vi "Sel_Insert QuickDrop.vi"(6 "Variant in":variant, 7 "Shift Pressed?":bool, 8 "error in (no error)":errorcluster, 10 "QD Combo Box Ref":refnum<vi>, 11 "QD Launch VI Ref":refnum<vi>) -> (0 "error out":errorcluster, 4 "Variant out":variant)   [LabVIEW 2014]
doc: "This quickdrop functionality will insert the selected node in the selected wire. Make sure that selected wire and node terminals have same data type.\n\nDefault Shortcut - [`]"
panel:
  in  "Undo Name":string="Quick Drop Keyboard Shortcut"
  # "Do not change the connector pane of this VI.\n\nSee the block diagram for directions on how to use this template."
  # "Specify the name of the Undo transaction"
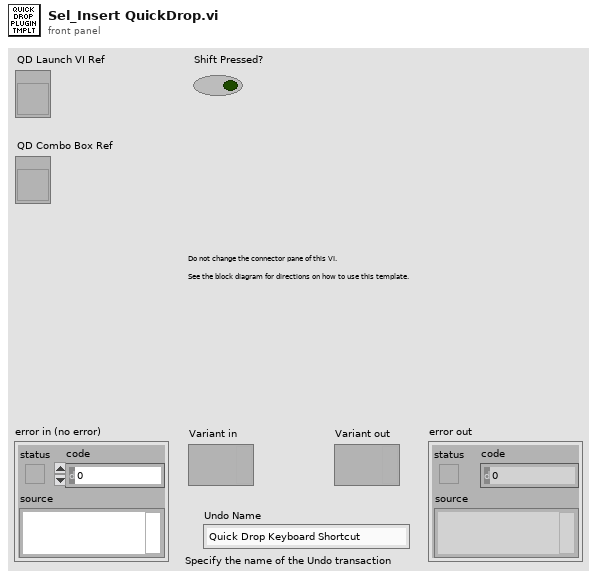
[diagram p1: front panel]
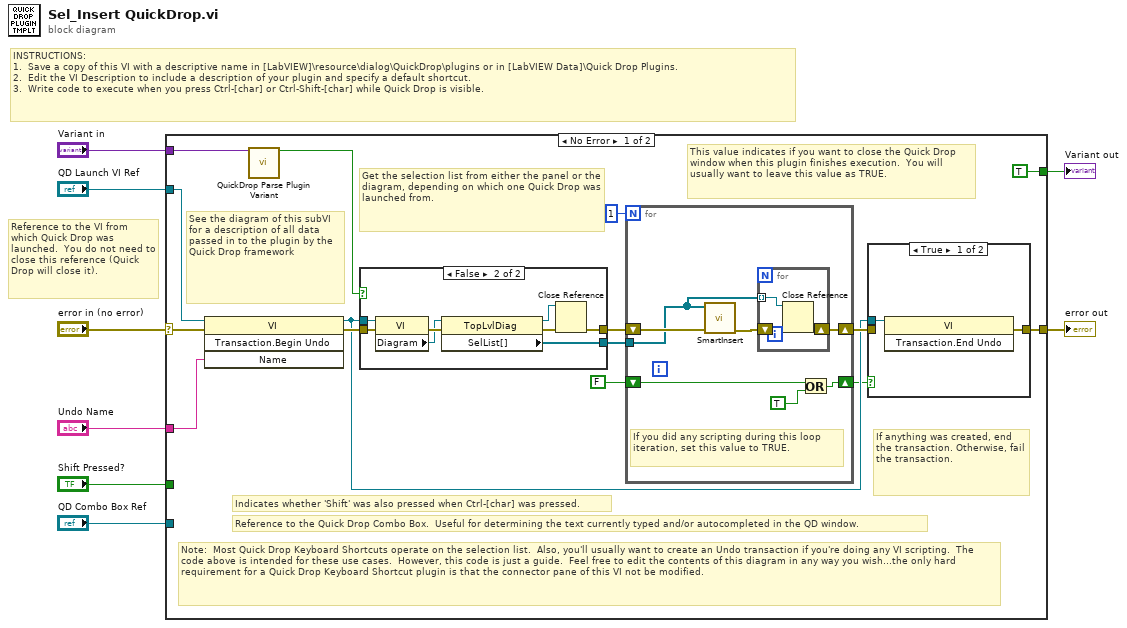
[diagram p0: block diagram]
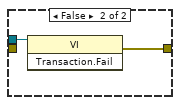
[diagram p2: hidden frame]
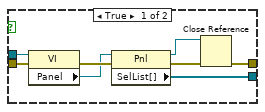
[diagram p3: hidden frame]
diagram:
  # "Reference to the VI from which Quick Drop was launched.  You do not need to close this reference (Quick Drop will close it)."
  # "INSTRUCTIONS:\n1.  Save a copy of this VI with a descriptive name in [LabVIEW]\\resource\\dialog\\QuickDrop\\plugins or in [LabVIEW Data]\\Quick Drop Plugins.\n2.  Edit the VI Description to include a description of your plugin and specify a default shortcut. \n3.  Write code to execute when you press Ctrl-[char] or Ctrl-Shift-[char] while Quick Drop is visible."
  n1 = case shown="No Error" "error in (no error)" {
    selector: "error in (no error)" -> [w22 w54]
    tunnel: [w16 w54] -> w7
    tunnel: "QD Launch VI Ref" -> [w21 _]
    tunnel: "Shift Pressed?" -> [_ _]
    tunnel: "QD Combo Box Ref" -> [_ _]
    tunnel: "Variant in" -> [w23 _]
    tunnel: "Undo Name" -> [w20 _]
    tunnel: [TRUE _] -> w1
    frame No Error {
      # "Note:  Most Quick Drop Keyboard Shortcuts operate on the selection list.  Also, you'll usually want to create an Undo transaction if you're doing any VI scripting.  The code above is intended for these use cases.  However, this code is just a guide.  Feel free to edit the contents of this diagram in any way you wish...the only hard requirement for a Quick Drop Keyboard Shortcut plugin is that the connector pane of this VI not be modified."
      # "Get the selection list from either the panel or the diagram, depending on which one Quick Drop was launched from."
      # "If anything was created, end the transaction. Otherwise, fail the transaction."
      # "This value indicates if you want to close the Quick Drop window when this plugin finishes execution.  You will usually want to leave this value as TRUE."
      # "See the diagram of this subVI for a description of all data passed in to the plugin by the Quick Drop framework"
      # "Reference to the Quick Drop Combo Box.  Useful for determining the text currently typed and/or autocompleted in the QD window."
      # "Indicates whether 'Shift' was also pressed when Ctrl-[char] was pressed."
      n2 = invoke class="VI" method="Transaction.Begin Undo"(reference=w21, error in=w22, "Name"=w20) -> (reference out=w13:refnum<vi>, error out=w17:errorcluster)  [unwired: 1 in, 2 out]
      n3 = call <vilib>:"QuickDrop Parse Plugin Variant.vi"("QDKS Variant in"=w23) -> ("QD Launch VI Panel?"=w18:bool)  [unwired: 12 in, 2 out]
      n4 = case shown="False" w18 {
        tunnel: w17 -> [w45 w53]
        tunnel: w13 -> [w44 w52]
        tunnel: [w39 w47] -> w15
        tunnel: [w38 w46] -> w10
        frame True {
          n5 = property class="VI"(reference=w44, error in=w45) -> (error out=w43:errorcluster, "Panel"=w42:refnum<vi>)  [unwired: 1 out]
          n6 = property class="Pnl"(reference=w42, error in=w43) -> (reference out=w40:refnum<vi>, error out=w41:errorcluster, "SelList[]"=w38:refnum<vi>[])
          n7 = Close Reference(reference=w40, error in (no error)=w41) -> (error out=w39:errorcluster)
        }
        frame False {
          n8 = property class="VI"(reference=w52, error in=w53) -> (error out=w51:errorcluster, "Diagram"=w50:refnum<vi>)  [unwired: 1 out]
          n9 = property class="TopLvlDiag"(reference=w50, error in=w51) -> (reference out=w48:refnum<vi>, error out=w49:errorcluster, "SelList[]"=w46:refnum<vi>[])
          n10 = Close Reference(reference=w48, error in (no error)=w49) -> (error out=w47:errorcluster)
        }
      }
      n11 = for {
        N: 1 -> [_]
        shift-right: [w27] -> w14
        shift-left: w15 -> [w26]
        shift-right: [w29] -> w11
        shift-left: FALSE -> [w30]
        tunnel: w10 -> [w24]
        # "If you did any scripting during this loop iteration, set this value to TRUE."
        n12 = call "SmartInsert.vi"("error in (no error)"=w26, "SelList[]"=w24) -> ("error out"=w25:errorcluster)  [unwired: 9 in]
        n13 = for {
          shift-right: [w33] -> w27
          shift-left: w25 -> [w32]
          tunnel: w24 -> [w31] mode=indexing
          n14 = Close Reference(reference=w31, error in (no error)=w32) -> (error out=w33:errorcluster)
        }
        n15 = Or(x=w30, y=TRUE ("x")) -> (x .or. y?=w29:bool)
      }
      n16 = case shown="True" w11 {
        tunnel: w13 -> [w34 w36]
        tunnel: [w35 w37] -> w16
        tunnel: w14 -> [_ _]
        frame True {
          n17 = invoke class="VI" method="Transaction.End Undo"(reference=w34) -> (error out=w35:errorcluster)  [unwired: 2 in, 2 out]
        }
        frame False {
          n18 = invoke class="VI" method="Transaction.Fail"(reference=w36) -> (error out=w37:errorcluster)  [unwired: 2 in, 2 out]
        }
      }
    }
    frame Error {
    }
  }
  "error out" <- w7
  "Variant out" <- w1
